vi "Evaluate.vi"(8 "error in (no error)":errorcluster, 11 "One In":refnum<class "Exactly.lvclass">) -> (0 "error out":errorcluster, 1 "Message":string, 2 "Passed?":bool)   [LabVIEW 2020, in "Exactly.lvlib" / "Exactly.lvclass"]
uses:
  Exactly.lvclass
  Exactly.lvclass/Exactly.ctl
  Core/VI Call/VI Call.lvclass
  Core/Comparator/Comparator.lvclass
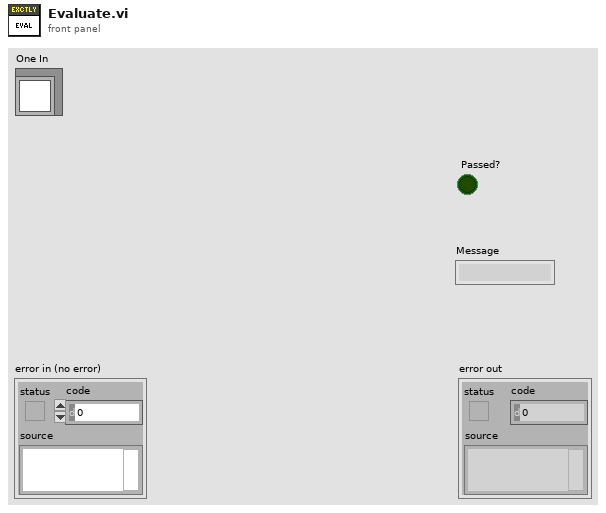
[diagram p1: front panel]
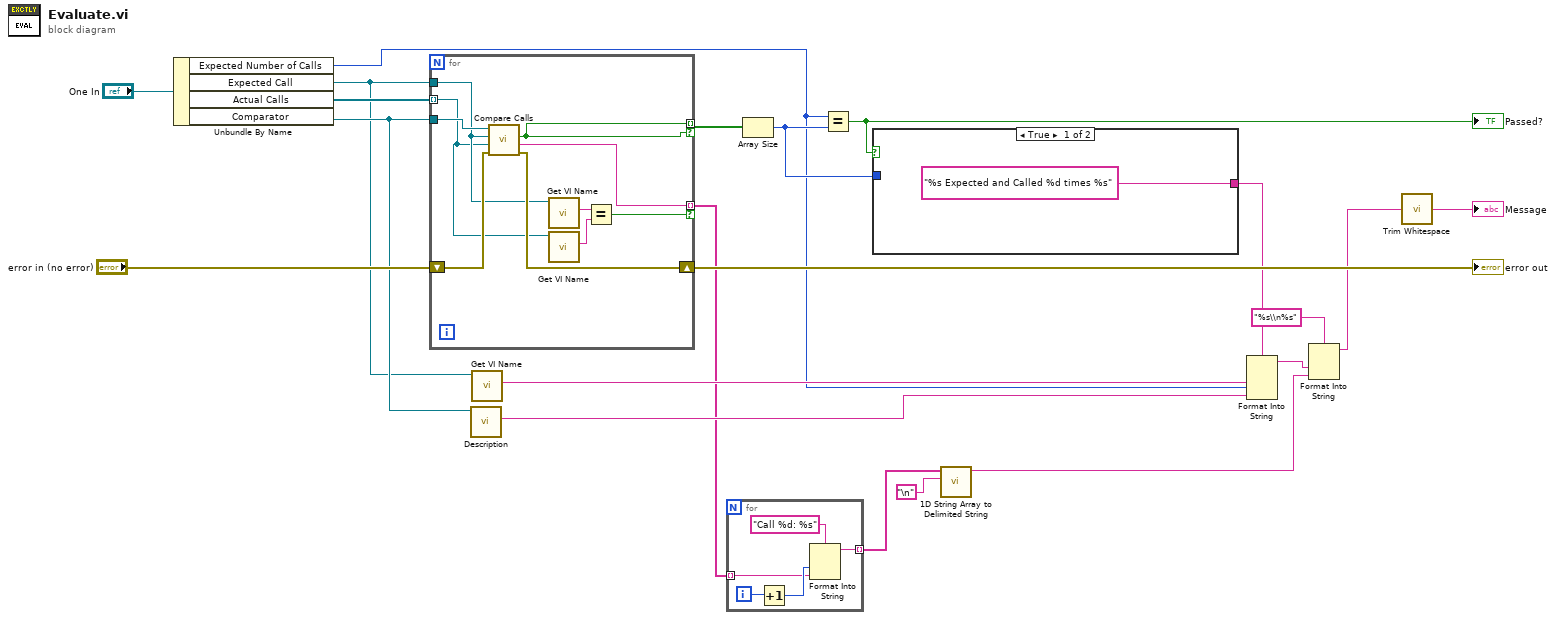
[diagram p0: block diagram]
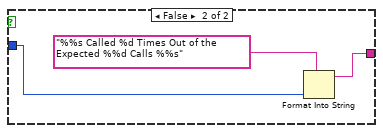
[diagram p2: hidden frame]
diagram:
  n1 = Unbundle By Name("One In") -> ("Expected Number of Calls"=w2:u32, "Expected Call"=w12:refnum<class "VI Call.lvclass">, "Actual Calls"=w19:refnum<class "VI Call.lvclass">[], "Comparator"=w16:refnum<class "Comparator.lvclass">)
  n2 = for {
    tunnel: w12 -> [w24]
    tunnel: w16 -> [w31]
    tunnel: w19 -> [w23] mode=indexing
    shift-right: [w29] -> w18
    shift-left: "error in (no error)" -> [w30]
    tunnel: [w28] -> w17 mode=indexing if=w28
    tunnel: [w27] -> w4 mode=indexing if=w22
    n3 = call-dynamic "Compare Calls.vi"("error in (no error)"=w30, "VI Call 2"=w23, "VI Call 1"=w24, "Comparator in"=w31) -> ("error out"=w29:errorcluster, "Description"=w27:string, "Equal?"=w28:bool)  [unwired: 5 in]
    n4 = call-dynamic "Get VI Name.vi"("VI Call In"=w24) -> ("VI Name"=w26:string)  [unwired: 10 in]
    n5 = call-dynamic "Get VI Name.vi"("VI Call In"=w23) -> ("VI Name"=w25:string)  [unwired: 10 in]
    n6 = Equal?(x=w26, y=w25) -> (x = y?=w22:bool)
  }
  "error out" <- w18
  n7 = call-dynamic "Description.vi"("Comparator in"=w16) -> ("Description"=w14:string)  [unwired: 9 in, 1 out]
  n8 = call-dynamic "Get VI Name.vi"("VI Call In"=w12) -> ("VI Name"=w11:string)  [unwired: 10 in]
  n9 = for {
    tunnel: w4 -> [w33] mode=indexing
    tunnel: [w32] -> w3 mode=indexing
    i -> [w35]
    n10 = Increment(x=w35) -> (x+1=w34:i32)
    n11 = Format Into String(format string="Call %d: %s", w34, w33) -> (resulting string=w32:string)  [unwired: 2 in, 1 out]
  }
  n12 = Array Size(array=w17) -> (size(s)=w13:i32)
  n13 = Equal?(x=w2, y=w13) -> (x = y?=w1:bool)
  "Passed?" <- w1
  n14 = case shown="True" w1 {
    tunnel: ["%s Expected and Called %d times %s" ("Message") w38] -> w15
    tunnel: w13 -> [_ w40]
    frame True {
    }
    frame False {
      n15 = Format Into String(format string="%%s Called %d Times Out of the Expected %%d Calls %%s" ("Message"), w40) -> (resulting string=w38:string)  [unwired: 2 in, 1 out]
    }
  }
  n16 = call <vilib>:"1D String Array to Delimited String.vi"("delimiter"="\n", "string array"=w3) -> ("delimited string"=w10:string)  [unwired: 9 in]
  n17 = Format Into String(format string=w15, w11, w2, w14) -> (resulting string=w9:string)  [unwired: 2 in, 1 out]
  n18 = Format Into String(format string="%s\\n%s", w9, w10) -> (resulting string=w7:string)  [unwired: 2 in, 1 out]
  n19 = call <vilib>:"Trim Whitespace.vi"("string"=w7) -> ("trimmed string"=→"Message":string)  [unwired: 1 in]
